vi "Scale.vi"(11 "Section Views in":refnum<class "Graph with Series View.lvclass">) -> (3 "Section Views out":refnum<class "Graph with Series View.lvclass">)   [LabVIEW 2025, in "Graph with Series View.lvclass"]
uses:
  Graph with Series View.lvclass
  Graph with Series View.lvclass/Graph with Series View.ctl
  Detail Graph/Graph with Section Views.lvclass
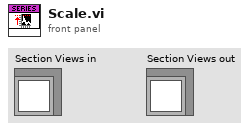
[diagram p1: front panel]
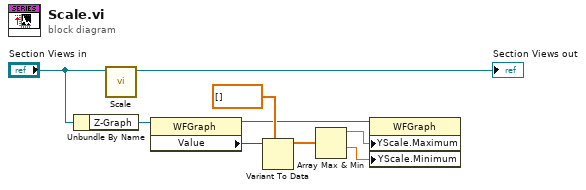
[diagram p0: block diagram]
diagram:
  n1 = Unbundle By Name("Section Views in") -> ("Z-Graph"=w7:refnum<vi>)
  n2 = call-parent "Scale.vi"("Section Views in"="Section Views in") -> ("Section Views out"=→"Section Views out":refnum<class "Graph with Series View.lvclass">)  [unwired: 10 in]
  n3 = property class="WFGraph"(reference=w7) -> (reference out=w3:refnum<vi>, "Value"=w6:variant)  [unwired: 1 in, 1 out]
  n4 = Variant To Data(type=dbl[] [], Variant=w6) -> (data=w4:dbl[])  [unwired: 1 in, 1 out]
  n5 = Array Max & Min(array=w4) -> (max value=w2:dbl, min value=w1:dbl)  [unwired: 2 out]
  n6 = property class="WFGraph"(reference=w3, "YScale.Maximum"=w2, "YScale.Minimum"=w1) -> ()  [unwired: 1 in, 2 out]
